vi "InitLabJack.vi"() -> (3 "LJConfig":T1={"Negative Channels 2"=[3, 5, 7, 9, 199, 199, 199, 199, 199, 199, 199], "Positive Channels 2"=[2, 4, 6, 8, 0, 1, 10, 11, 12, 13, 14], "Handle Out"=0, "error out"={"status"=FALSE, "code"=0, "source"=""}, "IO Types Out"=[]})   [LabVIEW 2023]
uses:
  TypeDefs/DataTypes/LabJackConfig.ctl
panel:
  in  "SettlingFactor":i32
  in  "Resolution":i32=12
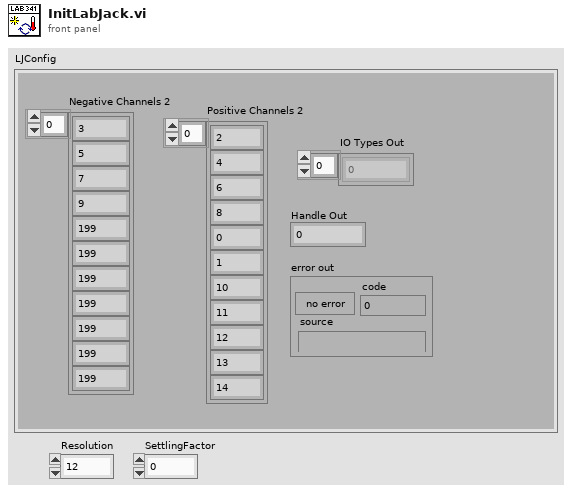
[diagram p1: front panel]
types:
  T1 = typedef "LabJackConfig.ctl" = cluster{"Negative Channels 2":i32[], "Positive Channels 2":i32[], "Handle Out":i32, "error out":errorcluster, "IO Types Out":i32[]}
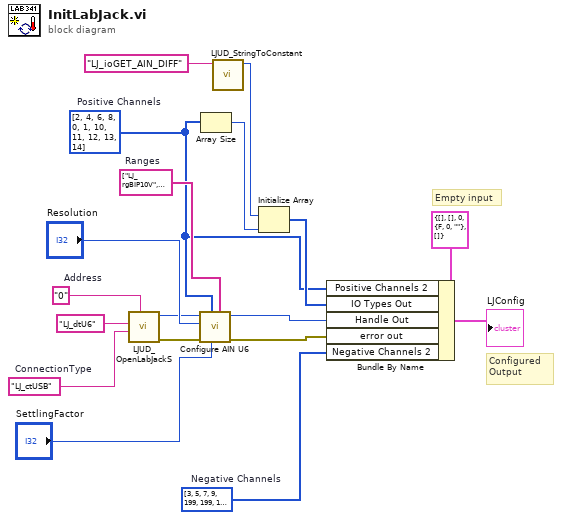
[diagram p0: block diagram]
diagram:
  w9 = i32[] [3, 5, 7, 9, 199, 199, 199, 199, 199, 199, 199]  # Negative Channels
  w17 = string[] ["LJ_rgBIP10V", "LJ_rgBIP10V", "LJ_rgBIP10V", "LJ_rgBIP10V", "LJ_rgBIP1V", "LJ_rgBIP1V", "LJ_rgBIP1V", "LJ_rgBIP1V", "LJ_rgBIP1V", "LJ_rgBIP1V", "LJ_rgBIP10V"]  # Ranges
  w8 = i32[] [2, 4, 6, 8, 0, 1, 10, 11, 12, 13, 14]  # Positive Channels
  w11 = "0"  # Address
  w13 = "LJ_ctUSB"  # ConnectionType
  # "Empty input"
  # "Configured \nOutput"
  n1 = call <vilib>:"LJUD_OpenLabJackS.vi"("Address"=w11, "ConnectionType"=w13, "DeviceType"="LJ_dtU6") -> ("error out"=w15:errorcluster, "Handle"=w14:i32)  [unwired: 6 in, 1 out]
  n2 = call <vilib>:"Configure AIN U6.vi"("Ranges"=w17, "SettlingFactor"="SettlingFactor", "Positive Channels"=w8, "error in"=w15, "Resolution"="Resolution", "Handle In"=w14) -> ("error out"=w4:errorcluster, "Handle Out"=w5:i32)  [unwired: 4 in]
  n3 = Array Size(array=w8) -> (size(s)=w18:i32)
  n4 = call <vilib>:"LJUD_StringToConstant.vi"("String"="LJ_ioGET_AIN_DIFF" ("IOType")) -> ("Constant Number"=w2:i32)  [unwired: 9 in, 1 out]
  n5 = Initialize Array(w2, w18) -> (w10:i32[])
  n6 = Bundle By Name(cluster=T1 {"Negative Channels 2"=[], "Positive Channels 2"=[], "Handle Out"=0, "error out"={"status"=FALSE, "code"=0, "source"=""}, "IO Types Out"=[]} ("LJConfig"), "Positive Channels 2"=w8, "IO Types Out"=w10, "Handle Out"=w5, "error out"=w4, "Negative Channels 2"=w9) -> (→"LJConfig":T1)
